vi "measure.vi"(11 "Qube":refnum<class "Qube.lvclass">) -> (0 "y":dbl, 1 "dy":dbl, 3 "Qube":refnum<class "Qube.lvclass">, 4 "counts":i32)   [LabVIEW 2017, in "Qube.lvclass"]
uses:
  Qube.lvclass
  <vilib>/Quanser/Rapid Control Prototyping Toolkit/hardware/HIL Board/HIL Read.vi
  <vilib>/Quanser/Rapid Control Prototyping Toolkit/hardware/HIL Board/HIL Board.lvclass
  <vilib>/Quanser/Rapid Control Prototyping Toolkit/hardware/HIL Board/_TypeSpecific/HIL Read Encoder (Scalar).vi
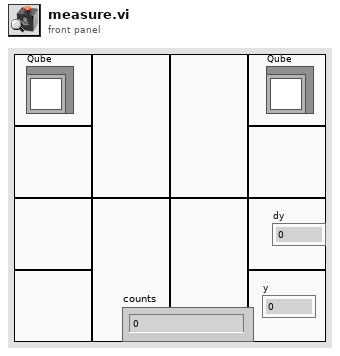
[diagram p1: front panel]
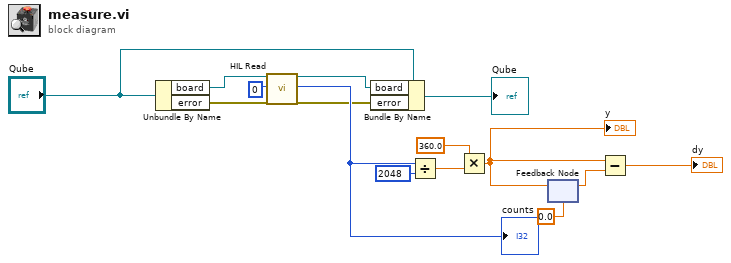
[diagram p0: block diagram]
diagram:
  n1 = Unbundle By Name("Qube") -> ("board"=w14:refnum<class "HIL Board.lvclass">, "error"=w15:errorcluster)
  n2 = call-poly "HIL Read"("board in"=w14, "channel"=u32 0, "error in (no error)"=w15) -> ("board out"=w9:refnum<class "HIL Board.lvclass">, "counts"=w13:i32, "error out"=w8:errorcluster)  [unwired: 14 in]
  "counts" <- w13
  n3 = Bundle By Name(cluster="Qube", "board"=w9, "error"=w8) -> (→"Qube":refnum<class "Qube.lvclass">)
  n4 = Divide(x=w13, y=2048) -> (x/y=w11:dbl)
  n5 = Multiply(x=360.0, y=w11) -> (x*y=w3:dbl)
  "y" <- w3
  n6 = feedback-in #1(w3) -> ()
  n7 = feedback #1(0.0) -> (w2:dbl)
  n8 = Subtract(x=w3, y=w2) -> (x-y=→"dy":dbl)
